vi "loopn.vi"() -> ()   [LabVIEW 2018, in "sandbox.lvlib"]
uses:
  sandbox.lvlib
panel:
  out "Numeric 2":i32
  out "Numeric":i32
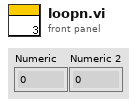
[diagram p1: front panel]
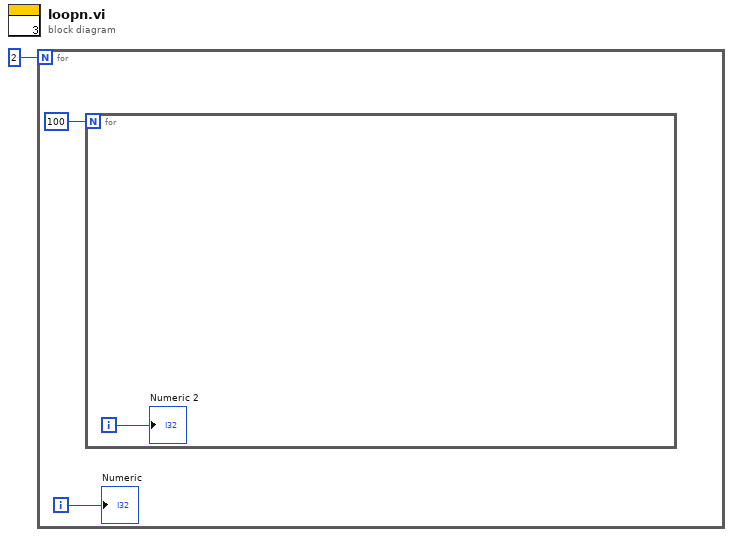
[diagram p0: block diagram]
diagram:
  n1 = for {
    N: 2 -> [_]
    i -> [w2]
    n2 = for {
      N: 100 -> [_]
      i -> [w4]
      "Numeric 2" <- w4
    }
    "Numeric" <- w2
  }
